vi "Apply.vi"(8 "error in (no error)":errorcluster, 11 "Read All CFG in":refnum<class "Read All CFG.lvclass">) -> (0 "error out":errorcluster, 3 "Read All CFG out":refnum<class "Read All CFG.lvclass">)   [LabVIEW 2024, in "NEO480HTA.lvlib" / "Read All CFG.lvclass"]
uses:
  Read All CFG.lvclass
  D:/git/HAL/HAL/Configurations/CFG JSON/CFG JSON.lvclass
  D:/git/HAL/HAL/Configurations/CFG Base/CFG Base.lvclass
  Configurations/CFG Base/CFG Base.lvclass/CFG Base.ctl
  7a8bdb5b-8155-4e79-b420-065c481765f3.vi
  d85a632b-e96c-4093-ba93-85e89de4a46d.vi
  8a89d08b-f2fd-4a62-ac40-9ffdf66b7b1b.vi
  557435a9-42a4-499c-b22b-c4a1f3a25359.vi
  <vilib>/JDP Science/JSONtext/Find Item.vi
  <vilib>/JDP Science/JSONtext/Next JSON Value.vi
  <vilib>/JDP Science/JSONtext/String Subset.vi
  <vilib>/JDP Science/JSONtext/Parsing/Advance past next JSON Value (inlined COPY).vi
  <vilib>/JDP Science/JSONtext/Parsing/Advance past whitespace.vi
  <vilib>/JDP Science/JSONtext/Parsing/Advance past String.vi
  <vilib>/JDP Science/JSONtext/Parsing/Advance past Number.vi
  <vilib>/JDP Science/JSONtext/Parsing/Advance past Line Ending.vi
  <vilib>/JDP Science/JSONtext/Parsing/Parse Full Path or Item Name.vi
  <vilib>/JDP Science/JSONtext/Parsing/Advance past Array.vi
  <vilib>/JDP Science/JSONtext/Parsing/Advance past Object.vi
  <vilib>/JDP Science/JSONtext/support/Error Cluster From Code.vi
  <vilib>/JDP Science/JSONtext/Offset/Find Item Locations by Path.vi
  <vilib>/JDP Science/JSONtext/JSON text to Variant.vi
  <vilib>/Utility/error.llb/Error Cluster From Error Code.vi
  <vilib>/xnet/xnet.llb/XNET Create Session (Frame Input Single-point).vi
  <vilib>/JDP Science/JSONtext/LVClass Serializer/JSONtext LVClass Serializer.lvclass
  <vilib>/ErrorRing/Error Ring.xnode
  <resource>/objmgr/xnet.rc
  CAN Interfaces/XNET/XNET Base CFG/XNET Base CFG.lvclass
  NEO480HTA.lvlib
  Configurations/CFG JSON/CFG JSON.lvclass
  Configurations/CFG Base/CFG Base.lvclass
panel:
  out "Interface:CAN:Termination":u32(ring)=1 items=["Off", "On"]
  out "Timing Type":u32(ring)=1 items=["Cyclic Data", "Event Data", "Cyclic Remote", "Event Remote"]
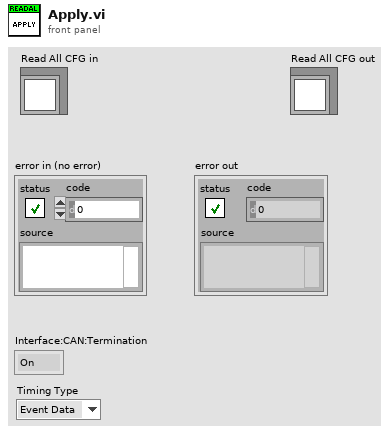
[diagram p1: front panel]
types:
  T1 = cluster{"Frame name":string, "Identifier":u32, "Payload Length":u32, "Timing Type":string, "Transmit Time":dbl, "Extended Identifier?":bool, "Comment":string}[]
  T2 = cluster{"Baud Rate":u32, "Comment":string, "Name":string}
  T3 = typedef "LVStringsAndValuesArrayTypeDef_U32.ctl" = cluster{"String":string, "Value":u32}[]
  T4 = cluster{"Frame name":string, "Identifier":u32, "Payload Length":u32, "Timing Type":u32, "Transmit Time":dbl, "Extended Identifier?":bool, "Comment":string}
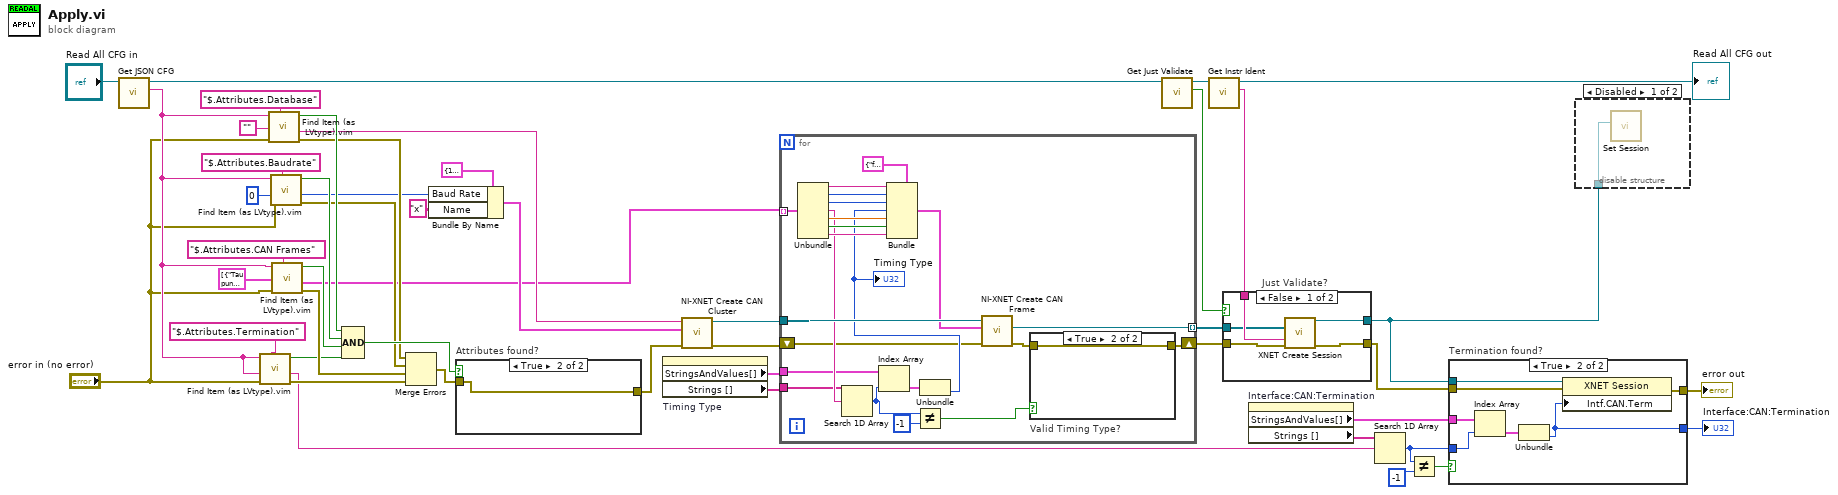
[diagram p0: block diagram]
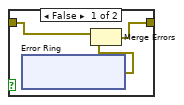
[diagram p3: hidden frame]
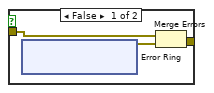
[diagram p4: hidden frame]
diagram:
  n1 = call "Get JSON CFG.vi"("CFG JSON in"="Read All CFG in") -> ("<JSON> CFG"=w15:string, "CFG JSON out"=w32:refnum<class "Read All CFG.lvclass">)  [unwired: 9 in]
  n2 = call "Find Item (as LVtype).vim"("$Path or Item Name"="$.Attributes.Termination", "error in (no error)"="error in (no error)", "Data Type and Default Value"=w15, "JSON"=w15) -> ("error out"=w29:errorcluster, "Data"=w18:string, "Found"=w30:bool)  [unwired: 4 in, 1 out]
  n3 = call "Find Item (as LVtype).vim"("$Path or Item Name"="$.Attributes.Database", "error in (no error)"="error in (no error)", "Data Type and Default Value"="", "JSON"=w15) -> ("error out"=w34:errorcluster, "Data"=w41:string, "Found"=w42:bool)  [unwired: 4 in, 1 out]
  n4 = call "Find Item (as LVtype).vim"("$Path or Item Name"="$.Attributes.Baudrate", "error in (no error)"="error in (no error)", "Data Type and Default Value"=u32 0, "JSON"=w15) -> ("error out"=w35:errorcluster, "Data"=w25:u32, "Found"=w45:bool)  [unwired: 4 in, 1 out]
  n5 = call "Find Item (as LVtype).vim"("$Path or Item Name"="$.Attributes.CAN Frames", "error in (no error)"="error in (no error)", "Data Type and Default Value"=T1 [{"Frame name"="Taupunkt", "Identifier"=1152, "Payload Length"=8, "Timing Type"="Event Data", "Transmit Time"=0.0, "Extended Identifier?"=FALSE, "Comment"=""}], "JSON"=w15) -> ("error out"=w36:errorcluster, "Data"=w21:T1, "Found"=w46:bool)  [unwired: 4 in, 1 out]
  n6 = Compound Arithmetic op=AND(w42, w45, w46, w30) -> (w44:bool)
  n7 = Merge Errors(w34, w35, w36, w29) -> (w37:errorcluster)
  n8 = Bundle By Name(cluster=T2 {"Baud Rate"=125000, "Comment"="", "Name"=""} ("CAN Cluster"), "Baud Rate"=w25, "Name"="x") -> (w24:T2)
  n9 = case "Attributes found?" shown="True" w44 {
    tunnel: w37 -> [w50 w57]
    tunnel: [w51 w57] -> w40
    frame False {
      n10 = xnode "Error Ring"() -> ("error out"=w49:errorcluster)
      n11 = Merge Errors(w50, w49) -> (w51:errorcluster)
    }
    frame True {
    }
  }
  n12 = property on="Timing Type" class="Ring (strict)"() -> ("StringsAndValues[]"=w5:T3, "Strings []"=w4:string[])  [unwired: 2 in, 2 out]
  n13 = call "NI-XNET Create CAN Cluster.vi"("error in"=w40, "CAN Cluster"=w24, "database in"=w41) -> ("error out"=w38:errorcluster, "cluster out"=w39:refnum<k21>)  [unwired: 7 in]
  n14 = for {
    tunnel: w39 -> [w79]
    shift-right: [w64] -> w33
    shift-left: w38 -> [w58]
    tunnel: [w78] -> w22 mode=indexing
    tunnel: w21 -> [w77] mode=indexing
    tunnel: w5 -> [w60]
    tunnel: w4 -> [w59]
    n15 = Unbundle(w77) -> ("Frame name"=w75:string, "Identifier"=w74:u32, "Payload Length"=w73:u32, "Timing Type"=w66:string, "Transmit Time"=w71:dbl, "Extended Identifier?"=w69:bool, "Comment"=w70:string)
    n16 = Search 1D Array(1D array=w59, element=w66) -> (index of element=w67:i32)  [unwired: 1 in]
    n17 = Index Array(array=w60, index=w67) -> (element=w68:cluster{"String":string, "Value":u32})
    n18 = Not Equal?(x=w67, y=-1) -> (x != y?=w62:bool)
    n19 = Unbundle(w68) -> ("Value"=w65:u32)  [unwired: 1 out]
    "Timing Type" <- w65
    n20 = Bundle(cluster=T4 {"Frame name"="frame1", "Identifier"=1, "Payload Length"=8, "Timing Type"=1, "Transmit Time"=0.0, "Extended Identifier?"=FALSE, "Comment"=""} ("CAN Frame"), "Frame name"=w75, "Identifier"=w74, "Payload Length"=w73, "Timing Type"=w65, "Transmit Time"=w71, "Extended Identifier?"=w69, "Comment"=w70) -> (w72:T4)
    n21 = call "NI-XNET Create CAN Frame.vi"("error in"=w58, "CAN Frame"=w72, "cluster in"=w79) -> ("error out"=w63:errorcluster, "frame out"=w78:refnum<k21>)  [unwired: 6 in, 1 out]
    n22 = case "Valid Timing Type?" shown="True" w62 {
      tunnel: w63 -> [w81 w88]
      tunnel: [w82 w88] -> w64
      frame False {
        n23 = xnode "Error Ring"() -> ("error out"=w80:errorcluster)
        n24 = Merge Errors(w81, w80) -> (w82:errorcluster)
      }
      frame True {
      }
    }
  }
  n25 = call "Get Just Validate.vi"("CFG Base in"=w32) -> ("Just Validate"=w3:bool, "CFG Base out"=w7:refnum<class "Read All CFG.lvclass">)  [unwired: 9 in]
  n26 = call-dynamic "Get Instr Ident.vi"("CFG JSON in"=w7) -> ("Instr Ident"=w16:string, "CFG JSON out"=→"Read All CFG out":refnum<class "Read All CFG.lvclass">)  [unwired: 8 in, 1 out]
  n27 = case "Just Validate?" shown="False" w3 {
    tunnel: w33 -> [w93 w94]
    tunnel: w22 -> [w90 _]
    tunnel: w16 -> [w92 _]
    tunnel: [w91 w94] -> w9
    tunnel: [w89 _] -> w6
    frame False {
      n28 = call-poly <vilib>:"XNET Create Session.vi"("frame list"=w90, "interface"=w92, "error in (no error)"=w93) -> ("session out"=w89:refnum<k21>, "error out"=w91:errorcluster)  [unwired: 11 out]
    }
    frame True {
    }
  }
  n29 = property on="Interface:CAN:Termination" class="Ring (strict)"() -> ("StringsAndValues[]"=w19:T3, "Strings []"=w20:string[])  [unwired: 2 in, 2 out]
  n30 = Search 1D Array(1D array=w20, element=w18) -> (index of element=w13:i32)  [unwired: 1 in]
  n31 = Not Equal?(x=w13, y=-1) -> (x != y?=w14:bool)
  n32 = case "Termination found?" shown="True" w14 {
    tunnel: w6 -> [_ w103]
    tunnel: [w95 w102] -> w28
    tunnel: w13 -> [w96 w100]
    tunnel: w19 -> [_ w99]
    tunnel: [w96 w98] -> w11
    tunnel: w9 -> [w95 w97]
    frame False {
    }
    frame True {
      n33 = Index Array(array=w99, index=w100) -> (element=w101:cluster{"String":string, "Value":u32})
      n34 = Unbundle(w101) -> ("Value"=w98:u32)  [unwired: 1 out]
      n35 = property class="XNET Session"(reference=w103, error in=w97, "Intf.CAN.Term"=w98) -> (error out=w102:errorcluster)  [unwired: 1 out]
    }
  }
  "error out" <- w28
  "Interface:CAN:Termination" <- w11
  n36 = disable-structure shown="Disabled" {
    disable-tunnel: w6 -> [w104 _]
    frame Disabled {
      n37 = call "Set Session.vi"("Session"=w104) -> ()  [unwired: 9 in, 2 out]
    }
    frame Enabled {
    }
  }
